vi "Begin.vi"(11 "Image Size":T1=enum."160x120") -> (0 "error out":errorcluster)   [LabVIEW 2011]
doc: "Called before other user functions, this VI is expected to open initial I/O refnums, load in file data, and do all program initialization. Notice that the <B>error out</B> terminal is simply used for data flow. Wiring it to other structures or subVIs ensures that this VI runs first."
uses:
  <vilib>/Rock Robotics/WPI/Camera/WPI_CameraImageSize.ctl
  <vilib>/Rock Robotics/WPI/Camera/WPI_CameraWhite Balance Values.ctl
  <vilib>/Rock Robotics/WPI/Camera/WPI_CameraExposure Values.ctl
  <vilib>/Rock Robotics/WPI/Camera/WPI_CameraFrameRate.ctl
  <vilib>/Rock Robotics/SystemInterfaces/DIO/FPGA_DIOPWMChannel.ctl
  <vilib>/Rock Robotics/WPI/Joystick/WPI_JoystickDeviceEnum.ctl
  <vilib>/Rock Robotics/SystemInterfaces/DIO/FPGA_DIOChannel.ctl
  <vilib>/Rock Robotics/SystemInterfaces/AI/FPGA_AIGyroChannel.ctl
  <vilib>/Rock Robotics/WPI/MotorControl/WPI_MotorControlOpen Victor.vi
  Robot Global Data.vi
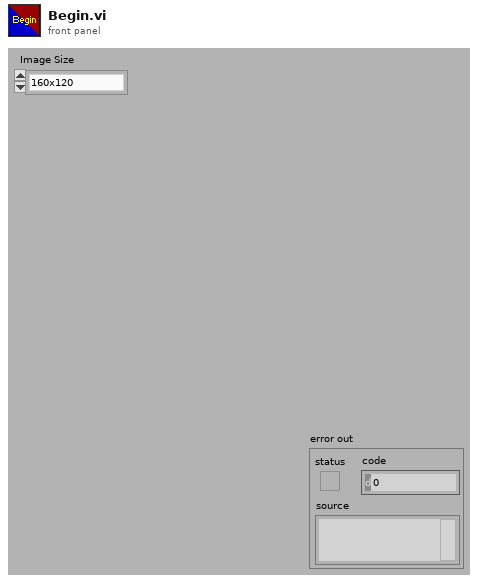
[diagram p1: front panel]
types:
  T1 = typedef "WPI_CameraImageSize.ctl" = enum16{"640x480", "320x240", "160x120"}
  T2 = typedef "FPGA_DIOPWMChannel.ctl" = enum8{"PWM 1", "PWM 2", "PWM 3", "PWM 4", "PWM 5", "PWM 6", "PWM 7", "PWM 8", "PWM 9", "PWM 10", "Invalid"}
  T3 = typedef "FPGA_AIGyroChannel.ctl" = enum8{"AI 1", "AI 2", "Invalid"}
  T4 = typedef "FPGA_DIOChannel.ctl" = enum8{"DIO 1", "DIO 2", "DIO 3", "DIO 4", "DIO 5", "DIO 6", "DIO 7", "DIO 8", "DIO 9", "DIO 10", "DIO 11", "DIO 12", "DIO 13", "DIO 14", "Invalid"}
  T5 = typedef "WPI_JoystickDeviceEnum.ctl" = enum16{"USB 1", "USB 2", "USB 3", "USB 4", "Kinect 1", "Kinect 2"}
  T6 = typedef "WPI_CameraFrameRate.ctl" = u32
  T7 = typedef "WPI_CameraExposure Values.ctl" = enum16{"Auto", "Flicker-free 50 Hz", "Flicker-free 60 Hz", "Hold current"}
  T8 = typedef "WPI_CameraWhite Balance Values.ctl" = enum16{"Auto", "Fixed indoor", "Fixed outdoor 1", "Fixed outdoor 2", "Fixed fluorescent 1", "Fixed fluorescent 2", "Hold current"}
  T9 = typedef "WPI_MotorControlDeviceRef.ctl" = cluster{"DeviceStatus":errorcluster, "Type":enum16{"PWM", "CAN"}, "PWM":cluster{"Digital Module":T10, "PWM Channel":T2, "DeadBand":T11}, "CAN":cluster{"Device Number":u8, "Control Mode":T12, "Semaphore":T13, "Max Vout":dbl}, "Invert":bool, "TransformRef":T14, "InvTransformRef":T14}
  T10 = typedef "FPGA_TypedefDigitalModule.ctl" = enum16{"Digital Module 1", "Digital Module 2"}
  T11 = typedef "WPI_PWMDeadband.ctl" = cluster{"Name":string, "maxPositivePwm":i32, "minPositivePwm":i32, "centerPwm":i32, "maxNegativePwm":i32, "minNegativePwm":i32, "angularRange":u16}
  T12 = typedef "WPI_CANJaguar_ControlMode.ctl" = enum8{"Percent VBus", "Current", "Speed", "Position", "Voltage"}
  T13 = typedef "Semaphore RefNum" = refnum<k1>
  T14 = typedef "WPI_PWMTransform_ConPane.ctl" = refnum<vi>
  T15 = typedef "WPI_CameraDevRef.ctl" = cluster{"Camera Address":string, "CameraStatus":errorcluster, "Acquire Image Notifier":refnum<notifier>}
  T16 = typedef "WPI_JoystickDevRef.ctl" = cluster{"Device":T5}
  T17 = typedef "WPI_ServoDeviceRef.ctl" = cluster{"DeviceStatus":errorcluster, "Digital Module":T10, "PWM Channel":T2, "DeadBand":T11}
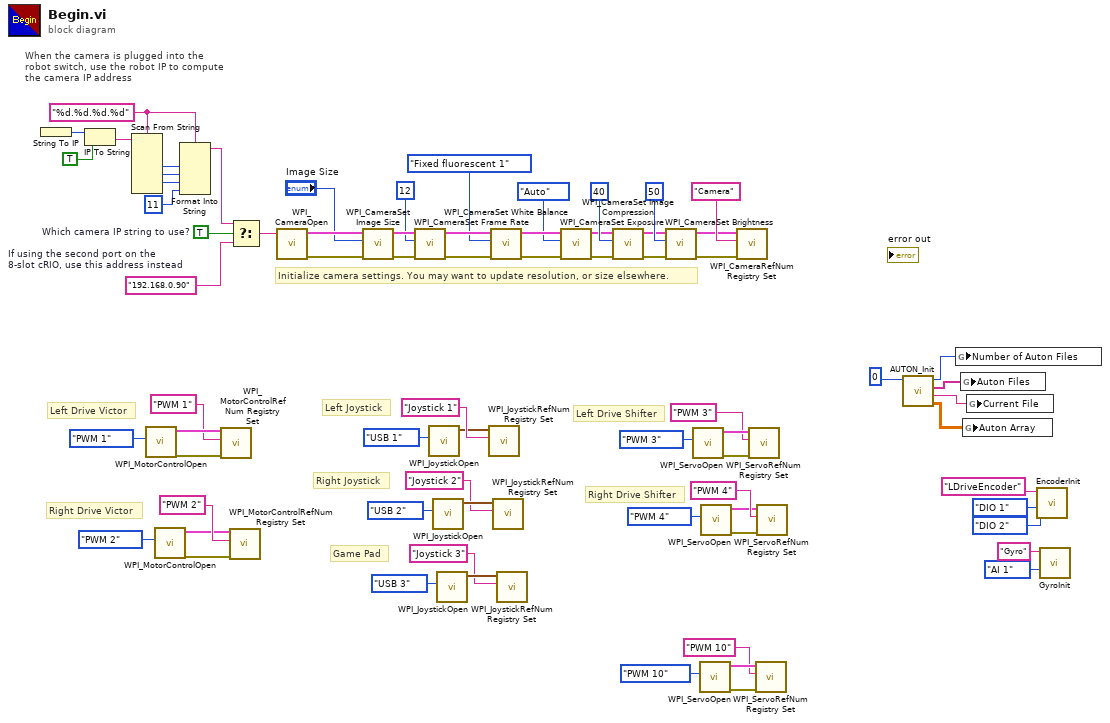
[diagram p0: block diagram]
diagram:
  w40 = TRUE  # Which camera IP string to use?
  w44 = "%d.%d.%d.%d" ("format string")
  w41 = "192.168.0.90"  # If using the second port on the 8-slot cRIO, use this address instead
  # "Right Drive Shifter"
  # "Left Drive Shifter"
  # "Right Joystick"
  # "Left Joystick"
  # "Game Pad"
  # "Right Drive Victor"
  # "Left Drive Victor"
  # "When the camera is plugged into the\nrobot switch, use the robot IP to compute\nthe camera IP address"
  # "Initialize camera settings. You may want to update resolution, or size elsewhere."
  n1 = String To IP() -> (0:w51:u32)  [unwired: 1 in]
  n2 = IP To String(1:TRUE ("dot notation? (F)"), 2:w51) -> (0:w49:string)
  n3 = Scan From String(format string=w44, input string=w49) -> (output 1=w48:i32, output 2=w47:i32, output 3=w46:i32)  [unwired: 7 in, 3 out]
  n4 = call-poly <vilib>:"WPI_MotorControlOpen.vi"("PWM Channel"=FPGA_DIOPWMChannel."PWM 1") -> ("error out"=w38:errorcluster, "MotorControlDeviceRef"=w39:T9)  [unwired: 9 in]
  n5 = call-poly <vilib>:"WPI_MotorControlOpen.vi"("PWM Channel"=FPGA_DIOPWMChannel."PWM 2") -> ("error out"=w33:errorcluster, "MotorControlDeviceRef"=w32:T9)  [unwired: 9 in]
  n6 = Format Into String(format string=w44, w48, w47, w46, 11 ("Compression")) -> (resulting string=w42:string)  [unwired: 2 in, 1 out]
  n7 = call <vilib>:"WPI_MotorControlRefNum Registry Set.vi"("error in (no error)"=w38, "refnum name"="PWM 1", "MotorControlDevRef"=w39) -> ()  [unwired: 7 in, 2 out]
  n8 = call <vilib>:"WPI_MotorControlRefNum Registry Set.vi"("error in (no error)"=w33, "refnum name"="PWM 2", "MotorControlDevRef"=w32) -> ()  [unwired: 7 in, 2 out]
  n9 = Select(t=w42, s=w40, f=w41) -> (s? t:f=w43:string)
  n10 = call <vilib>:"WPI_CameraOpen.vi"("Camera Address"=w43) -> ("error out"=w63:errorcluster, "CameraDevRef"=w64:T15)  [unwired: 1 in, 8 out]
  n11 = call <vilib>:"WPI_CameraSet Image Size.vi"("error in (no error)"=w63, "Image Size"="Image Size", "CameraDevRef"=w64) -> ("error out"=w62:errorcluster, "CameraDevRef Out"=w65:T15)  [unwired: 7 out]
  n12 = call <vilib>:"WPI_CameraSet Frame Rate.vi"("error in (no error)"=w62, "Frame Rate (fps)"=T6 12, "CameraDevRef"=w65) -> ("error out"=w61:errorcluster, "CameraDevRef Out"=w67:T15)  [unwired: 7 out]
  n13 = call <vilib>:"WPI_JoystickOpen.vi"("JoystickDevice"=WPI_JoystickDeviceEnum."USB 1") -> ("JoystickDevRef"=w23:T16)  [unwired: 10 in]
  n14 = call <vilib>:"WPI_JoystickOpen.vi"("JoystickDevice"=WPI_JoystickDeviceEnum."USB 2") -> ("JoystickDevRef"=w28:T16)  [unwired: 10 in]
  n15 = call <vilib>:"WPI_JoystickOpen.vi"("JoystickDevice"=WPI_JoystickDeviceEnum."USB 3") -> ("JoystickDevRef"=w31:T16)  [unwired: 10 in]
  n16 = call <vilib>:"WPI_JoystickRefNum Registry Set.vi"("refnum name"="Joystick 1", "JoystickDevRef"=w23) -> ()  [unwired: 8 in, 2 out]
  n17 = call <vilib>:"WPI_CameraSet White Balance.vi"("error in (no error)"=w61, "White Balance"=WPI_CameraWhite_Balance_Values."Fixed fluorescent 1", "CameraDevRef"=w67) -> ("error out"=w60:errorcluster, "CameraDevRef Out"=w66:T15)  [unwired: 7 out]
  n18 = call <vilib>:"WPI_JoystickRefNum Registry Set.vi"("refnum name"="Joystick 2", "JoystickDevRef"=w28) -> ()  [unwired: 8 in, 2 out]
  n19 = call <vilib>:"WPI_JoystickRefNum Registry Set.vi"("refnum name"="Joystick 3", "JoystickDevRef"=w31) -> ()  [unwired: 8 in, 2 out]
  n20 = call <vilib>:"WPI_CameraSet Exposure.vi"("error in (no error)"=w60, "Exposure"=WPI_CameraExposure_Values."Auto", "CameraDevRef"=w66) -> ("error out"=w59:errorcluster, "CameraDevRef Out"=w69:T15)  [unwired: 7 out]
  n21 = call <vilib>:"WPI_CameraSet Image Compression.vi"("error in (no error)"=w59, "Compression"=40, "CameraDevRef"=w69) -> ("error out"=w58:errorcluster, "CameraDevRef Out"=w68:T15)  [unwired: 7 out]
  n22 = call <vilib>:"WPI_CameraSet Brightness.vi"("error in (no error)"=w58, "Brightness"=50, "CameraDevRef"=w68) -> ("error out"=w56:errorcluster, "CameraDevRef Out"=w57:T15)  [unwired: 7 out]
  n23 = call <vilib>:"WPI_ServoOpen.vi"("PWM Channel"=FPGA_DIOPWMChannel."PWM 3") -> ("error out"=w22:errorcluster, "ServoDeviceRef"=w21:T17)  [unwired: 9 in]
  n24 = call <vilib>:"WPI_ServoOpen.vi"("PWM Channel"=FPGA_DIOPWMChannel."PWM 10") -> ("error out"=w4:errorcluster, "ServoDeviceRef"=w3:T17)  [unwired: 9 in]
  n25 = call <vilib>:"WPI_ServoOpen.vi"("PWM Channel"=FPGA_DIOPWMChannel."PWM 4") -> ("error out"=w15:errorcluster, "ServoDeviceRef"=w16:T17)  [unwired: 9 in]
  n26 = call <vilib>:"WPI_CameraRefNum Registry Set.vi"("error in (no error)"=w56, "refnum name"="Camera", "CameraDevRef"=w57) -> ()  [unwired: 9 out]
  n27 = call <vilib>:"WPI_ServoRefNum Registry Set.vi"("error in (no error)"=w22, "refnum name"="PWM 3", "ServoDeviceRef"=w21) -> ()  [unwired: 7 in, 2 out]
  n28 = call <vilib>:"WPI_ServoRefNum Registry Set.vi"("error in (no error)"=w4, "refnum name"="PWM 10", "ServoDeviceRef"=w3) -> ()  [unwired: 7 in, 2 out]
  n29 = call <vilib>:"WPI_ServoRefNum Registry Set.vi"("error in (no error)"=w15, "refnum name"="PWM 4", "ServoDeviceRef"=w16) -> ()  [unwired: 7 in, 2 out]
  n30 = call "AUTON_Init.vi"("Default File"=0) -> ("Auton Array"=w12:dbl[][], "Current File"=w11:string, "Auton Files"=w13:string[], "Number of Auton Files"=w14:i64)  [unwired: 7 in]
  n31 = global write "Robot Global Data.vi" "Number of Auton Files"(w14) -> ()
  n32 = global write "Robot Global Data.vi" "Auton Files"(w13) -> ()
  n33 = global write "Robot Global Data.vi" "Auton Array"(w12) -> ()
  n34 = global write "Robot Global Data.vi" "Current File"(w11) -> ()
  n35 = call "EncoderInit.vi"("refnum name"="LDriveEncoder", "DIO Channel"=FPGA_DIOChannel."DIO 1", "DIO Channel 2"=FPGA_DIOChannel."DIO 2") -> ()  [unwired: 8 in]
  n36 = call "GyroInit.vi"("refnum name"="Gyro", "Analog Channel"=FPGA_AIGyroChannel."AI 1") -> ()  [unwired: 8 in]
